vi "Write Current Slide.vi"(8 "error in (no error)":errorcluster, 10 "Current Slide":i32, 11 "Parse Presentation in":refnum<class "Parse Presentation.lvclass">) -> (0 "error out":errorcluster, 3 "Parse Presentation out":refnum<class "Parse Presentation.lvclass">)   [LabVIEW 2015, in "Parse Presentation.lvclass"]
uses:
  Parse Presentation.lvclass
  Parse Presentation.lvclass/Parse Presentation.ctl
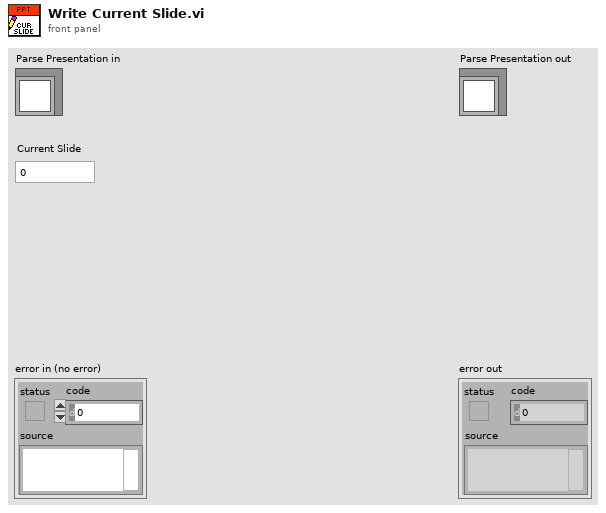
[diagram p1: front panel]
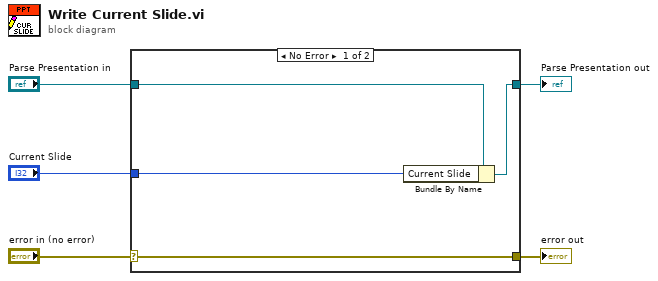
[diagram p0: block diagram]
diagram:
  n1 = case shown="No Error" "error in (no error)" {
    selector: "error in (no error)" -> [w9 w10]
    tunnel: [w9 w10] -> w4
    tunnel: [w7 w11] -> w2
    tunnel: "Parse Presentation in" -> [w8 w11]
    tunnel: "Current Slide" -> [w6 _]
    frame No Error {
      n2 = Bundle By Name(cluster=w8, "Current Slide"=w6) -> (w7:refnum<class "Parse Presentation.lvclass">)
    }
    frame Error {
    }
  }
  "error out" <- w4
  "Parse Presentation out" <- w2
